vi "Status LEDs.vi"(8 "Array Error":bool[](array[boolean]), 9 "Array Aktiv":bool[](array[boolean]), 11 "Array LED":refnum<vi>[](array[refnum])) -> ()   [LabVIEW 2020, in "Backup.lvlib"]
uses:
  Backup.lvlib
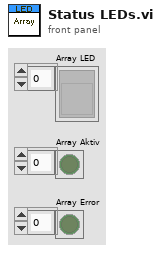
[diagram p1: front panel]
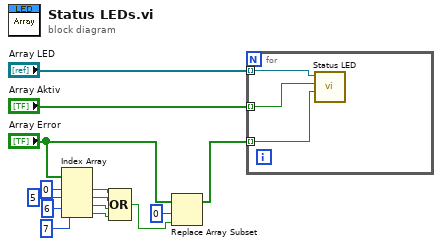
[diagram p0: block diagram]
diagram:
  n1 = Index Array(array="Array Error", index #1=0 ("Index"), index #2=5 ("Index"), index #3=6 ("Index"), index #4=7 ("Index")) -> (element #1=w7:bool, element #2=w6:bool, element #3=w5:bool, element #4=w4:bool)
  n2 = Compound Arithmetic op=OR ("Mehrfacharithmetik")(w7, w6, w5, w4) -> (w2:bool)
  n3 = Replace Array Subset(array="Array Error", new element=w2, index=0 ("Index")) -> (w1:bool[])
  n4 = for {
    tunnel: "Array Aktiv" -> [w16] mode=indexing
    tunnel: "Array LED" -> [w17] mode=indexing
    tunnel: w1 -> [w15] mode=indexing
    n5 = call "Status LED.vi"("Fehler"=w15, "Aktiv"=w16, "Boolean (Eingang)"=w17) -> ()  [unwired: 9 in]
  }
